vi "Defer Panel Updates.vi"() -> ()   [LabVIEW 2012]
panel:
  in  "Defer Panel Updates":bool
  in  "Stop Button":bool
  in  "Disabled State":T1(ring)
  out "Waveform Chart 2":dbl(graph)
  in  "Thermometer 2":dbl(slide) scale=0.0..100.0
  in  "Vertical Fill Slide 2":dbl(slide) scale=0.0..10.0
  in  "Pause Button 2":bool
  in  "Eject Button 2":bool
  in  "Help Button 2":bool
  in  "Down Button 2":bool
  in  "Copy Button 2":bool
  in  "Play Button 2":bool
  in  "Mail Button 2":bool
  in  "Open Button 2":bool
  in  "Add Button 2":bool
  in  "New Button 2":bool
  in  "Up Button 2":bool
  in  "OK Button 2":bool
  out "Waveform Chart":dbl(graph)
  in  "Thermometer":dbl(slide) scale=0.0..100.0
  in  "Vertical Fill Slide":dbl(slide) scale=0.0..10.0
  in  "Pause Button":bool
  in  "Eject Button":bool
  in  "Help Button":bool
  in  "Down Button":bool
  in  "Copy Button":bool
  in  "Play Button":bool
  in  "Mail Button":bool
  in  "Open Button":bool
  in  "Add Button":bool
  in  "New Button":bool
  in  "Up Button":bool
  in  "OK Button":bool
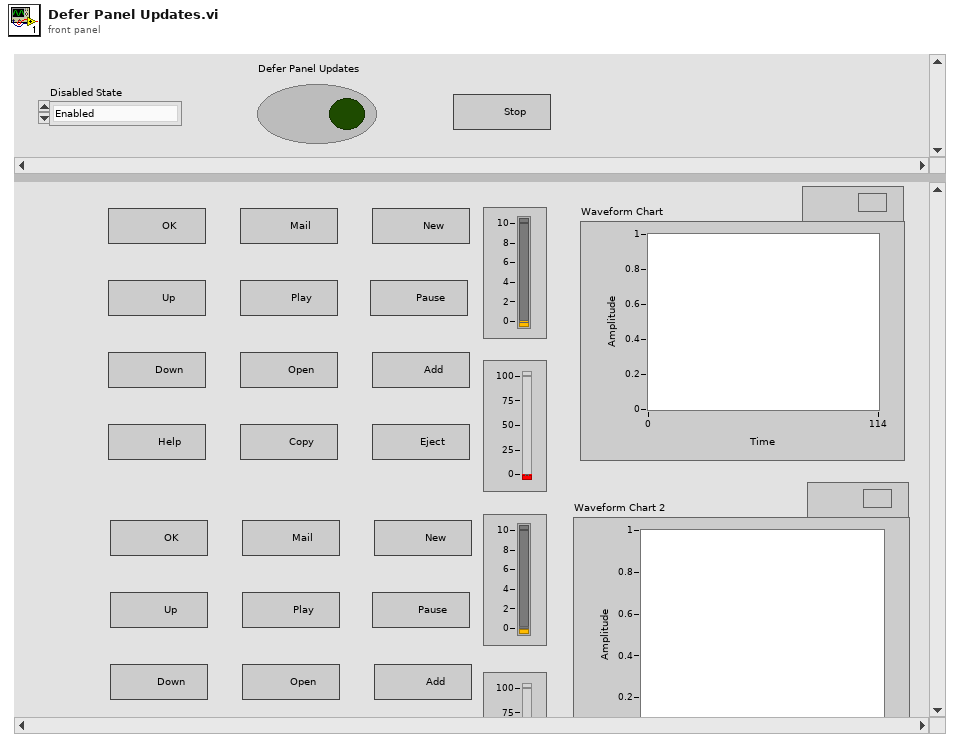
[diagram p1: front panel]
types:
  T1 = enum8{"Enabled", "Disabled", "Disabled and Grayed Out"}
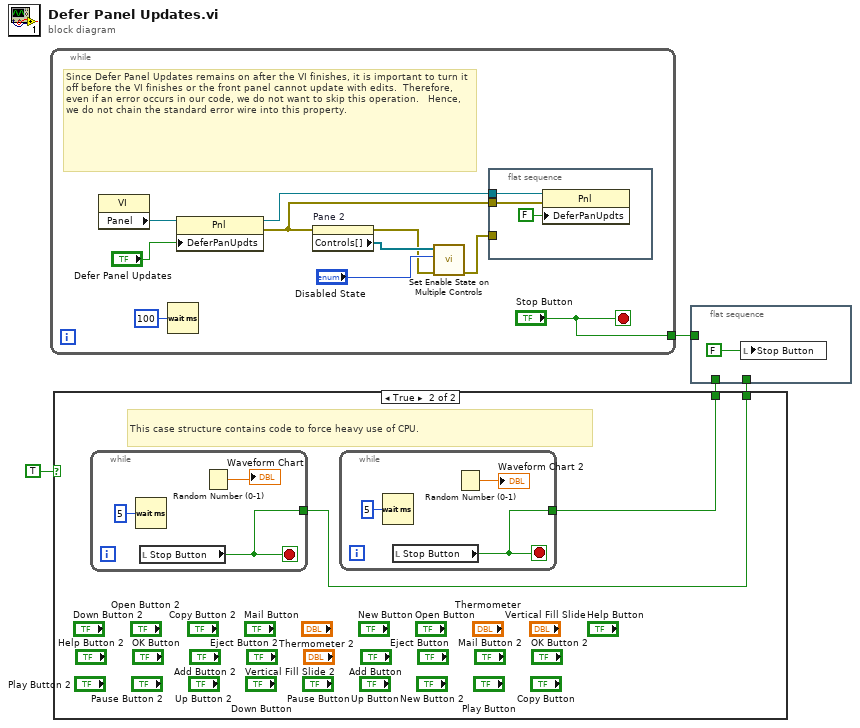
[diagram p0: block diagram]
diagram:
  n1 = while {
    tunnel: ["Stop Button"] -> w4
    stop <- "Stop Button" stop-if-true
    # "Since Defer Panel Updates remains on after the VI finishes, it is important to turn it off before the VI finishes or the front panel cannot update with edits.  Therefore, even if an error occurs in our code, we do not want to skip this operation.   Hence, we do not chain the standard error wire into this property."
    n2 = property class="VI"() -> ("Panel"=w8:refnum<vi>)  [unwired: 2 in, 2 out]
    n3 = Wait (ms)(milliseconds to wait=u32 100) -> ()  [unwired: 1 out]
    n4 = property class="Pnl"(reference=w8, "DeferPanUpdts"="Defer Panel Updates") -> (reference out=w7:refnum<vi>, error out=w10:errorcluster)  [unwired: 1 in]
    n5 = property on="Pane 2" class="Pane"(error in=w10) -> (error out=w11:errorcluster, "Controls[]"=w12:refnum<vi>[])  [unwired: 1 in, 1 out]
    n6 = call "Set Enable State on Multiple Controls.vi"("Error In"=w11, "Disabled State"="Disabled State", "Controls"=w12) -> ("Error Out"=w9:errorcluster)  [unwired: 8 in]
    n7 = flat-sequence {
      tunnel: w10 -> [w16]
      tunnel: w9 -> [_]
      tunnel: w7 -> [w15]
      frame #0 {
        n8 = property class="Pnl"(reference=w15, error in=w16, "DeferPanUpdts"=FALSE ("Defer Panel Updates")) -> ()  [unwired: 2 out]
      }
    }
  }
  n9 = case shown="True" TRUE {
    tunnel: [_ w19] -> w2
    tunnel: [_ w18] -> w1
    frame False {
    }
    frame True {
      # "This case structure contains code to force heavy use of CPU."
      n10 = while {
        tunnel: [w25] -> w18
        stop <- w25 stop-if-true
        n11 = Wait (ms)(milliseconds to wait=u32 5) -> ()  [unwired: 1 out]
        n12 = local read "Stop Button"() -> (w25:bool)
        n13 = Random Number (0-1)() -> (number: 0 to 1=→"Waveform Chart":dbl)
      }
      n14 = while {
        tunnel: [w22] -> w19
        stop <- w22 stop-if-true
        n15 = Wait (ms)(milliseconds to wait=u32 5) -> ()  [unwired: 1 out]
        n16 = local read "Stop Button"() -> (w22:bool)
        n17 = Random Number (0-1)() -> (number: 0 to 1=→"Waveform Chart 2":dbl)
      }
    }
  }
  n18 = flat-sequence {
    tunnel: w4 -> [_]
    tunnel: w2 -> [_]
    tunnel: w1 -> [_]
    frame #0 {
      n19 = local write "Stop Button"(FALSE ("Stop Button")) -> ()
    }
  }
